vi "Pre-Init.vi"(8 "error in (no error)":errorcluster, 11 "Red Pitaya Digitizer in":refnum<class "Red Pitaya Digitizer.lvclass">) -> (0 "error out":errorcluster, 3 "Red Pitaya Digitizer out":refnum<class "Red Pitaya Digitizer.lvclass">)   [LabVIEW 2021, in "Red Pitaya Digitizer.lvclass"]
uses:
  Red Pitaya Digitizer.lvclass
  Red Pitaya Digitizer.lvclass/Red Pitaya Digitizer.ctl
  Instruments/Pulse Driver/Pulse Driver.lvclass
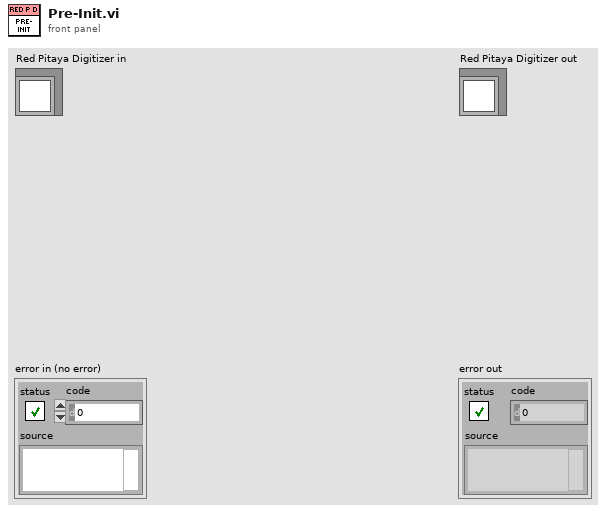
[diagram p1: front panel]
types:
  T1 = typedef "Pusle Driver Configuration.ctl" = cluster{"Post-trigger delay":dbl, "Post-trigger duration":dbl, "Rate":dbl, "Ranges":dbl[], "Re-name channels":string[], "Active channels":string, "External clock":bool}
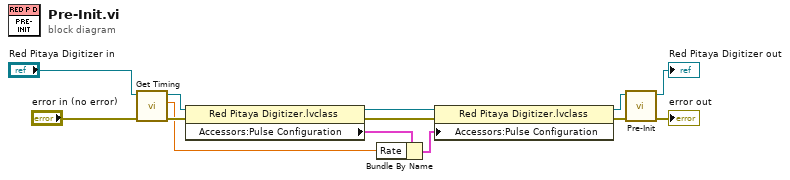
[diagram p0: block diagram]
diagram:
  n1 = call-dynamic "Get Timing.vi"("error in (no error)"="error in (no error)", "Red Pitaya Digitizer in"="Red Pitaya Digitizer in") -> ("error out"=w9:errorcluster, "Rate"=w1:dbl, "Red Pitaya Digitizer out"=w7:refnum<class "Red Pitaya Digitizer.lvclass">)  [unwired: 6 in, 1 out]
  n2 = property class="Red Pitaya Digitizer.lvclass"(reference=w7, error in=w9) -> (reference out=w5:refnum<class "Red Pitaya Digitizer.lvclass">, error out=w8:errorcluster, "Accessors:Pulse Configuration"=w3:T1)
  n3 = Bundle By Name(cluster=w3, "Rate"=w1) -> (w2:T1)
  n4 = property class="Red Pitaya Digitizer.lvclass"(reference=w5, error in=w8, "Accessors:Pulse Configuration"=w2) -> (reference out=w4:refnum<class "Red Pitaya Digitizer.lvclass">, error out=w6:errorcluster)
  n5 = call-parent "Pre-Init.vi"("error in (no error)"=w6, "Pulse Driver in"=w4) -> ("error out"=→"error out":errorcluster, "Pulse Driver out"=→"Red Pitaya Digitizer out":refnum<class "Red Pitaya Digitizer.lvclass">)  [unwired: 8 in]
